vi "Close.vi"(8 "error in":errorcluster, 11 "Reply Protocol DataSocket in":refnum<class "Reply Protocol DataSocket.lvclass">) -> (0 "error out":errorcluster, 3 "Reply Protocol DataSocket out":refnum<class "Reply Protocol DataSocket.lvclass">)   [LabVIEW 2023, in "HAL GOOP4.lvlib" / "Reply Protocol DataSocket.lvclass"]
uses:
  Reply Protocol DataSocket.lvclass
  Reply Protocol DataSocket.lvclass/Reply Protocol DataSocket.ctl
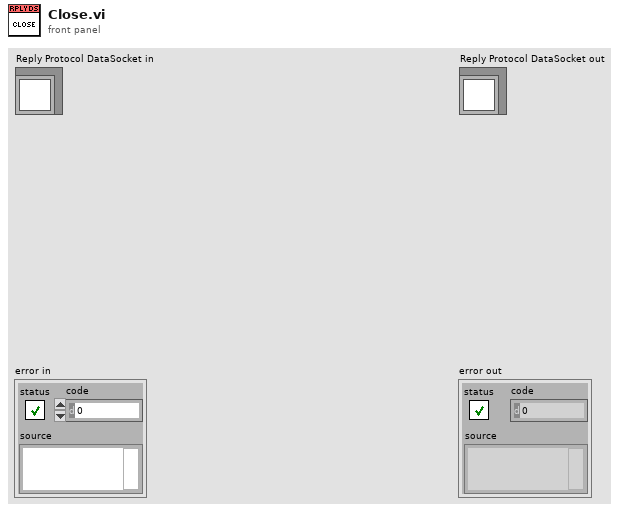
[diagram p1: front panel]
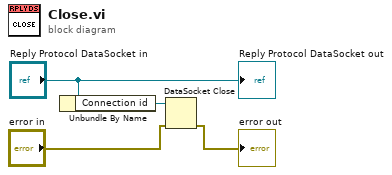
[diagram p0: block diagram]
diagram:
  n1 = Unbundle By Name("Reply Protocol DataSocket in") -> ("Connection id"=w4:refnum<k13>)
  n2 = DataSocket Close(8:"error in", 11:w4) -> (0:→"error out":errorcluster)  [unwired: 1 in, 1 out]
  "Reply Protocol DataSocket out" <- "Reply Protocol DataSocket in"
